vi "startup.vi"   [LabVIEW 2019]
doc: "Starts up and runs the main control program, splash screens, etc."
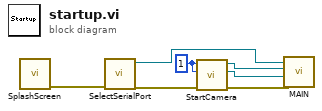
[diagram p0: block diagram]
diagram:
  w6 = u32 1 ("Gain")
  n1 = call "SplashScreen.vi"() -> ("Error Out"=w7:errorcluster)  [unwired: 11 in]
  n2 = call "SelectSerialPort.vi"("Error In"=w7) -> ("Error Out"=w5:errorcluster, "MotorController out"=w4:refnum<class "MotorController.lvclass">)  [unwired: 9 in]
  n3 = call "StartCamera.vi"("Error In"=w5, "ExposureTime_us"=w6, "Gain"=w6) -> ("Error Out"=w1:errorcluster, "TLCamera reference out"=w2:refnum<k24>, "TLCameraSDK reference out"=w3:refnum<k24>)  [unwired: 6 in]
  n4 = call "MAIN.vi"("Error In"=w1, "TLCamera reference out"=w2, "TLCameraSDK reference out"=w3, "MotorController out"=w4) -> ()  [unwired: 8 in]
